vi "TEST - File Exists - Array.vi"(8 "error in (no error)":errorcluster) -> (0 "error out":errorcluster, 2 "pass":bool)   [LabVIEW 2020]
uses:
  <userlib>/_OpenG.lib/error/error.llb/openg_error.lvlib
  source/library/openg_file.lvlib
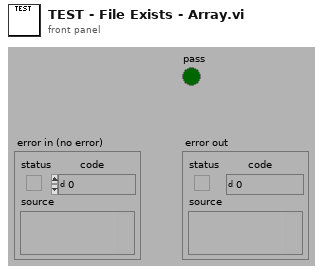
[diagram p1: front panel]
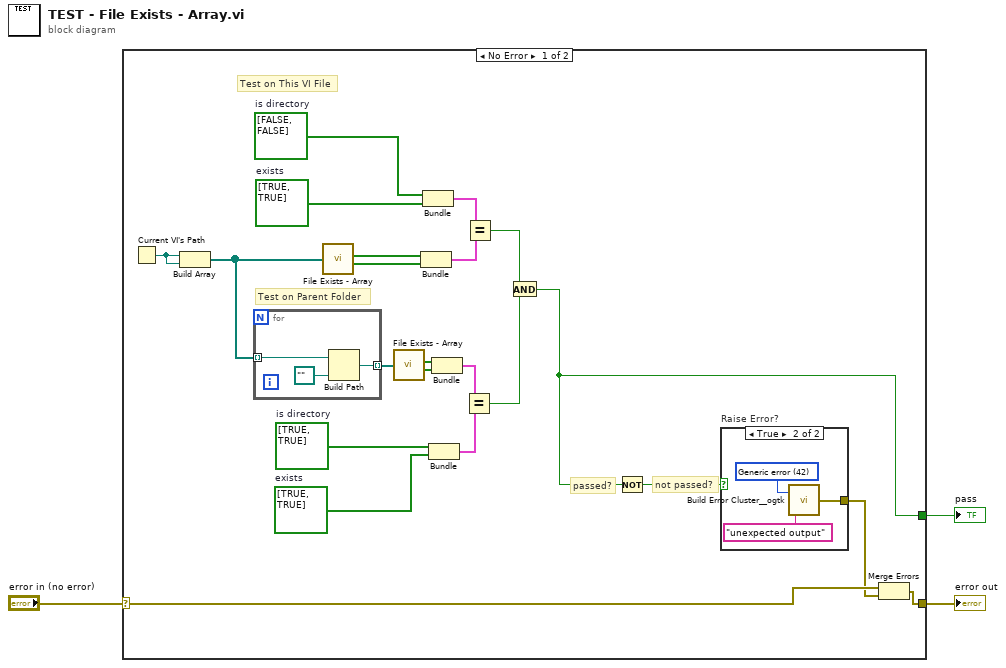
[diagram p0: block diagram]
diagram:
  n1 = case shown="No Error" "error in (no error)" {
    selector: "error in (no error)" -> [w25 w32]
    tunnel: [w10 _] -> w3
    tunnel: [w24 w32] -> w1
    frame No Error {
      w4 = bool[] [TRUE, TRUE]  # exists
      w5 = bool[] [FALSE, FALSE]  # is directory
      w6 = bool[] [TRUE, TRUE]  # exists
      w7 = bool[] [TRUE, TRUE]  # is directory
      # "Test on Parent Folder"
      # "Test on This VI File"
      # "not passed?"
      # "passed?"
      n2 = Current VI's Path() -> (path=w9:path)
      n3 = Build Array(w9, w9) -> (w8:path[])
      n4 = for {
        tunnel: [w27] -> w14 mode=indexing
        tunnel: w8 -> [w26] mode=indexing
        n5 = Build Path(base path=w26, name or relative path=path ".." ("path")) -> (appended path=w27:path)
      }
      n6 = call "File Exists - Array.vi"("file paths"=w8) -> ("is directory"=w21:bool[], "exists"=w20:bool[])  [unwired: 6 in]
      n7 = call "File Exists - Array.vi"("file paths"=w14) -> ("is directory"=w15:bool[], "exists"=w16:bool[])  [unwired: 6 in]
      n8 = Bundle("is directory"=w21, "exists"=w20) -> (w18:cluster{"is directory":bool[], "exists":bool[]})  [unwired: 1 in]
      n9 = Bundle("is directory"=w5, "exists"=w4) -> (w19:cluster{"is directory":bool[], "exists":bool[]})  [unwired: 1 in]
      n10 = Bundle("is directory"=w7, "exists"=w6) -> (w13:cluster{"is directory":bool[], "exists":bool[]})  [unwired: 1 in]
      n11 = Bundle("is directory"=w15, "exists"=w16) -> (w12:cluster{"is directory":bool[], "exists":bool[]})  [unwired: 1 in]
      n12 = Equal?(x=w12, y=w13) -> (x = y?=w11:bool)
      n13 = Equal?(x=w19, y=w18) -> (x = y?=w17:bool)
      n14 = And(x=w17, y=w11) -> (x .and. y?=w10:bool)
      n15 = Not(x=w10) -> (.not. x?=w22:bool)
      n16 = case "Raise Error?" shown="True" w22 {
        tunnel: [_ w29] -> w23
        frame False {
        }
        frame True {
          w30 = 42 items=["No error", "Argument error", "Memory is full", "Out of zone", "End of file", "File already open", "Generic file I/O error", "File not found", "File permission error", "Disk is full", "Duplicate path", "Too many files open", "System feature not enabled", "Resource file not found", "Cannot add resource", "Resource not found", "Image not found", "Image memory error", "Pen does not exist", "Config type invalid", "Config token not found", "Config parse error", "Config memory error", "Bad external code format", "Bad external code offset", "External code not present", "Null window", "Destroy window error", "Null menu", "Print aborted", "Bad print record", "Print driver error", "Windows error during printing", "Memory error during printing", "Print dialog error", "Generic print error", "Invalid device refnum", "Device not found", "Device parameter error", "Device unit error", "Cannot open device", "Device call aborted", "Generic error", "Cancelled by user", "Object ID too low", "Object ID too high", "Object not in heap", "Unknown heap", "Unknown object (invalid DefProc)", "Unknown object (DefProc not in table)", "Message out of range", "Invalid (null) method", "Unknown message", "Manager call not supported", "Bad address", "Network operation in progress", "Network operation timed out", "Connection is busy", "Network attribute not supported", "Network error", "Address in use", "System out of memory", "Connection aborted", "Connection refused", "Not connected", "Already connected", "Connection closed", "Initialization error (interapplication manager)", "Bad occurrence", "Wait on unbound occurrence handler", "Occurrence queue overflow", "Datalog type conflict", "Unused", "Unrecognized type (interapplication manager)", "Memory corrupt", "Failed to make temporary DLL", "Old CIN version", "Drag socket not found", "Failed to load drop-object", "Failed to register OLE object", "Failed to release OLE object", "Format specifier type mismatch", "Unknown format specifier", "Too few format specifiers", "Too many format specifiers", "Scan failed", "Newer CIN version", "Error converting to variant", "Runtime menu error", "Password tampered", "Variant attribute not found", "Incompatible variant data type", "Event data is not available", "Event Store is not present", "Occurrence is not found", "Event Queue is not created", "Event info is not available", "Refnum passed is NULL", "Error retrieving Class GUID", "Error retrieving CoClass GUID", "Error retrieving TypeLib GUID.", "Bad built application magic bytes.", "Specific driver is different from the specific driver associated with the Logical Name.", "There is no session opened to the class driver.", "Max Error", "MAX - Error with config objects", "MAX - Error loading configuration", "MAX - Group not supported"]
          n17 = call <userlib>:"Build Error Cluster__ogtk.vi"("String to Prepend to source (\"\")"="unexpected output" ("String to Prepend to source (\"\")"), "code"=w30) -> ("error out"=w29:errorcluster)
        }
      }
      n18 = Merge Errors(w25, w23) -> (w24:errorcluster)
    }
    frame Error {
    }
  }
  "pass" <- w3
  "error out" <- w1
